vi "Set Active Binding Post.vi"(8 "error in (no error)":errorcluster, 10 "Current Output Post (0: Normal)":u32(ring) items=["Normal", "AUX", "IB5725"], 11 "VISA resource name":refnum<visa-resource-name>) -> (0 "error out":errorcluster, 3 "VISA resource name out":refnum<visa-resource-name>)   [LabVIEW 2013, in "Fluke 5XXX Series Multicalibrators.lvlib"]
doc: "This VI selects the binding posts for current output. Once set, the calibrator retains the current post setting during power-off periods.\n\nNote:\n\nThis VI is available only for instrument models 5700A and 5720A."
uses:
  Fluke 5XXX Series Multicalibrators.lvlib
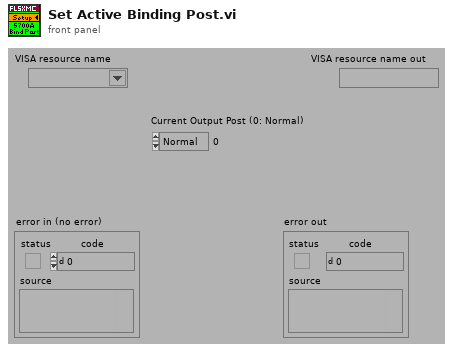
[diagram p1: front panel]
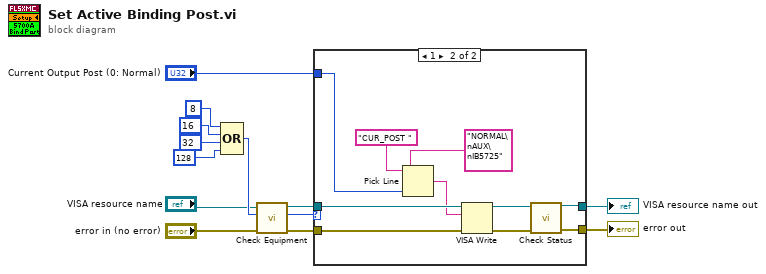
[diagram p0: block diagram]
diagram:
  n1 = Compound Arithmetic op=OR(8 ("Numeric"), 16 ("Numeric"), 32 ("Numeric"), 128 ("Numeric")) -> (w10:i32)
  n2 = call "Check Equipment.vi"("error in (no error)"="error in (no error)", "Bit Mask"=w10, "VISA resource name"="VISA resource name") -> ("error out"=w13:errorcluster, "Present?"=w12:u32, "VISA resource name out"=w11:refnum<visa-resource-name>)  [unwired: 6 in]
  n3 = case shown="1" w12 {
    tunnel: "Current Output Post (0: Normal)" -> [_ w20]
    tunnel: [w14 w16] -> w3
    tunnel: w13 -> [w15 w23]
    tunnel: w11 -> [w14 w22]
    tunnel: [w15 w19] -> w4
    frame 0, Default {
    }
    frame 1 {
      n4 = Pick Line(string ("")="CUR_POST " ("Reset Command"), multi-line string="NORMAL\nAUX\nIB5725", line index=w20) -> (output string=w21:string)
      n5 = VISA Write(VISA resource name=w22, write buffer=w21, error in (no error)=w23) -> (VISA resource name out=w17:refnum<visa-resource-name>, error out=w18:errorcluster)  [unwired: 1 out]
      n6 = call "Check Status.vi"("VISA resource name"=w17, "error in (no error)"=w18) -> ("VISA resource name out"=w16:refnum<visa-resource-name>, "error out"=w19:errorcluster)  [unwired: 12 in]
    }
  }
  "VISA resource name out" <- w3
  "error out" <- w4
